vi "LCP Get Volume Unit.vi"(8 "error in (no error)":errorcluster caption="Fehler (Eingang, kein Fehler)", 11 "Pump Handle":i64) -> (0 "error out":errorcluster caption="Fehler (Ausgang)", 2 "Volume Unit":i32, 3 "Prefix":i32)   [LabVIEW 2021, in "labbCAN_Pump_API.lvlib"]
doc: "LCP_Func long LCP_CALL LCP_GetVolumeUnit(dev_hdl hPump,\n int* pPrefix,\n int* pVolumeUnit);"
uses:
  labbCAN_Pump_API.lvlib
  labbCAN_Pump_API.dll
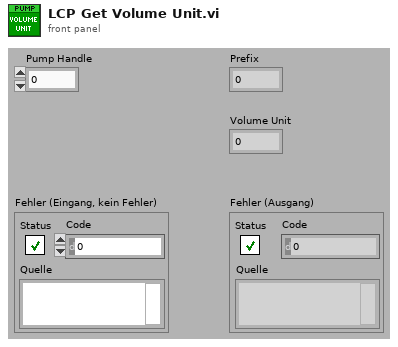
[diagram p1: front panel]
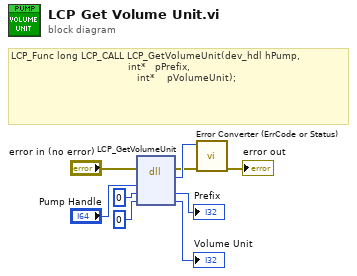
[diagram p0: block diagram]
diagram:
  # "LCP_Func long LCP_CALL LCP_GetVolumeUnit(dev_hdl hPump,\n\t                                      int*   pPrefix,\n                                          int*    pVolumeUnit);"
  n1 = dll-call lib="C:/Users/olaja/AppData/Local/CETONI_SDK/labbCAN_Pump_API.*" fn="LCP_GetVolumeUnit"(error in="error in (no error)", "hPump"="Pump Handle", "pPrefix"=0, "pVolumeUnit"=0) -> (error out=w2:errorcluster, "Rückgabetyp"=w3:i32, "pPrefix"=→"Prefix":i32, "pVolumeUnit"=→"Volume Unit":i32)  [unwired: 3 in, 1 out]
  n2 = call "Error Converter (ErrCode or Status).vi"("error in (no error)"=w2, "error code"=w3) -> ("error out"=→"error out":errorcluster)  [unwired: 9 in]
